vi "7-t-dist.vi"(0 "p_LW":T1, 5 "t":dbl, 11 "error in":errorcluster caption="err in") -> (2 "R(t)":dbl, 3 "La (t)":dbl, 4 "p_LW":T1, 6 "t":dbl, 8 "f (t)":dbl, 10 "F (t)":dbl, 15 "error out":errorcluster caption="err out")   [LabVIEW 2010, in "lv_02.lvlib"]
uses:
  p_5E7_LW.ctl
  lv_02.lvlib
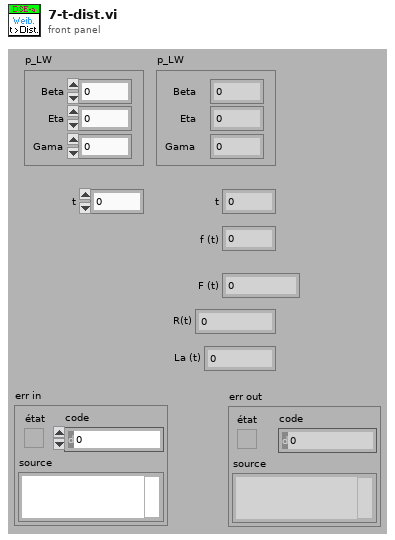
[diagram p1: front panel]
types:
  T1 = typedef "lv_02.lvlib/p_5E7_LW.ctl" = cluster{"Beta":dbl, "Eta":dbl, "Gama":dbl}
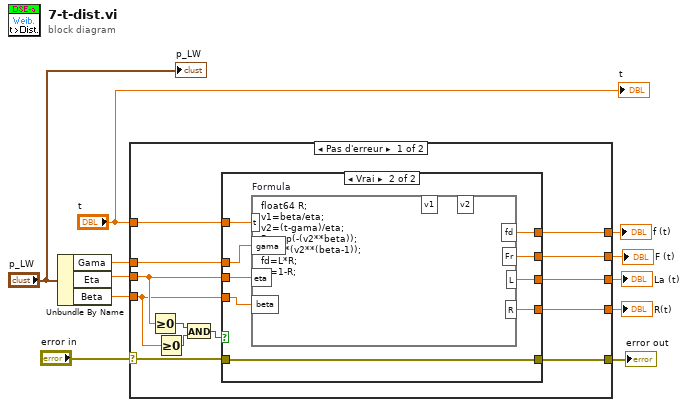
[diagram p0: block diagram]
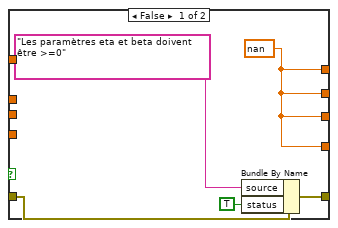
[diagram p2: hidden frame]
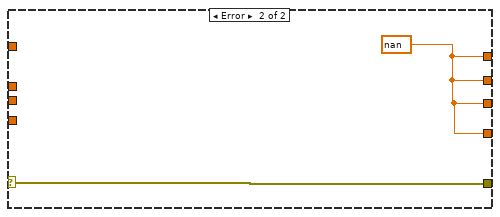
[diagram p3: hidden frame]
diagram:
  n1 = Unbundle By Name("p_LW") -> ("Gama"=w8:dbl, "Eta"=w5:dbl, "Beta"=w6:dbl)
  n2 = case shown="Pas d'erreur" "error in" {
    selector: "error in" -> [w21 w40]
    tunnel: "t" -> [w24 _]
    tunnel: [w23 w39] -> w10
    tunnel: w8 -> [w22 _]
    tunnel: w6 -> [w16 _]
    tunnel: w5 -> [w17 _]
    tunnel: [w20 w40] -> w4
    tunnel: [w19 w39] -> w3
    tunnel: [w18 w39] -> w2
    tunnel: [w15 w39] -> w1
    frame No Error {
      n3 = Greater Or Equal To 0?(x=w17) -> (x >= 0?=w14:bool)
      n4 = Greater Or Equal To 0?(x=w16) -> (x >= 0?=w13:bool)
      n5 = And(x=w14, y=w13) -> (x .and. y?=w12:bool)
      n6 = case shown="Vrai" w12 {
        tunnel: w24 -> [_ w37]
        tunnel: [w25 w33] -> w23
        tunnel: w22 -> [_ w36]
        tunnel: w16 -> [_ w31]
        tunnel: w17 -> [_ w35]
        tunnel: w21 -> [w29 w38]
        tunnel: [w26 w38] -> w20
        tunnel: [w25 w32] -> w19
        tunnel: [w25 w34] -> w18
        tunnel: [w25 w30] -> w15
        frame False {
          w25 = nan
          n7 = Bundle By Name(cluster=w29, "source"="Les paramètres eta et beta doivent  être >=0", "status"=TRUE) -> (w26:errorcluster)
        }
        frame True {
          n8 = formula code="float64 R;\nv1=beta/eta;\nv2=(t-gama)/eta;\nR=exp(-(v2**beta));\nL=v1*(v2**(beta-1));\nfd=L*R;\nFr=1-R;"("t"=w37, "gama"=w36, "eta"=w35, "beta"=w31) -> ("R"=w34:dbl, "L"=w33:dbl, "fd"=w30:dbl, "Fr"=w32:dbl)  [unwired: 2 out]
        }
      }
    }
    frame Error {
      w39 = nan
    }
  }
  "La (t)" <- w10
  "error out" <- w4
  "F (t)" <- w3
  "R(t)" <- w2
  "f (t)" <- w1
  "t" <- "t"
  "p_LW" <- "p_LW"
